vi "LVClass_SlopesPostProcessList dtor.vi"(0 "SlopesPostProcessorList in":refnum<class "SlopesPostProcessorList.lvclass">, 11 "error in (no error)":errorcluster) -> (4 "SlopesPostProcessorList out":refnum<class "SlopesPostProcessorList.lvclass">, 15 "error out":errorcluster)   [LabVIEW 2020, in "SlopesPostProcessorList.lvclass"]
doc: "SlopesPostProcessorList destructor.\n\n--------------------------------------------------------------------------------\n\n<B>SlopesPostProcessorListIn </B> : SlopesPostProcessorList object.\n<B>SlopesPostProcessorListOut </B> : SlopesPostProcessorList object.\n<B>ErrorIn </B> : Error\n<B>ErrorOut </B> : Error\n\n--------------------------------------------------------------------------------"
uses:
  SlopesPostProcessorList.lvclass
  SlopesPostProcessorList.lvclass/SlopesPostProcessorList.ctl
  HasoSlopes.lvclass
  Pupil.lvclass
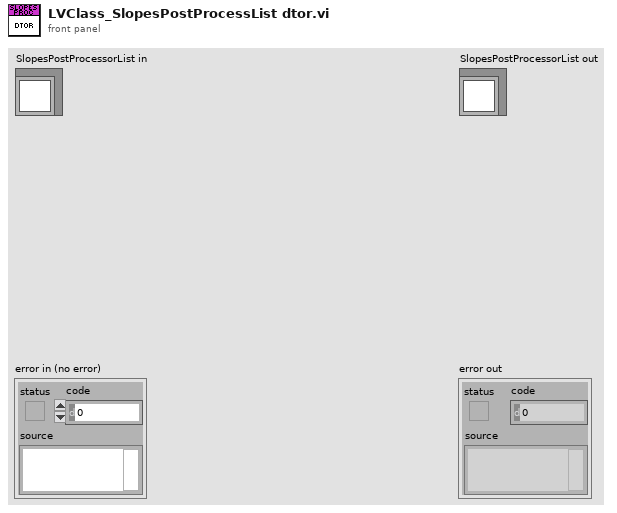
[diagram p1: front panel]
types:
  T1 = typedef "Handle creation.ctl" = enum16{"By ctor", "By write function"}
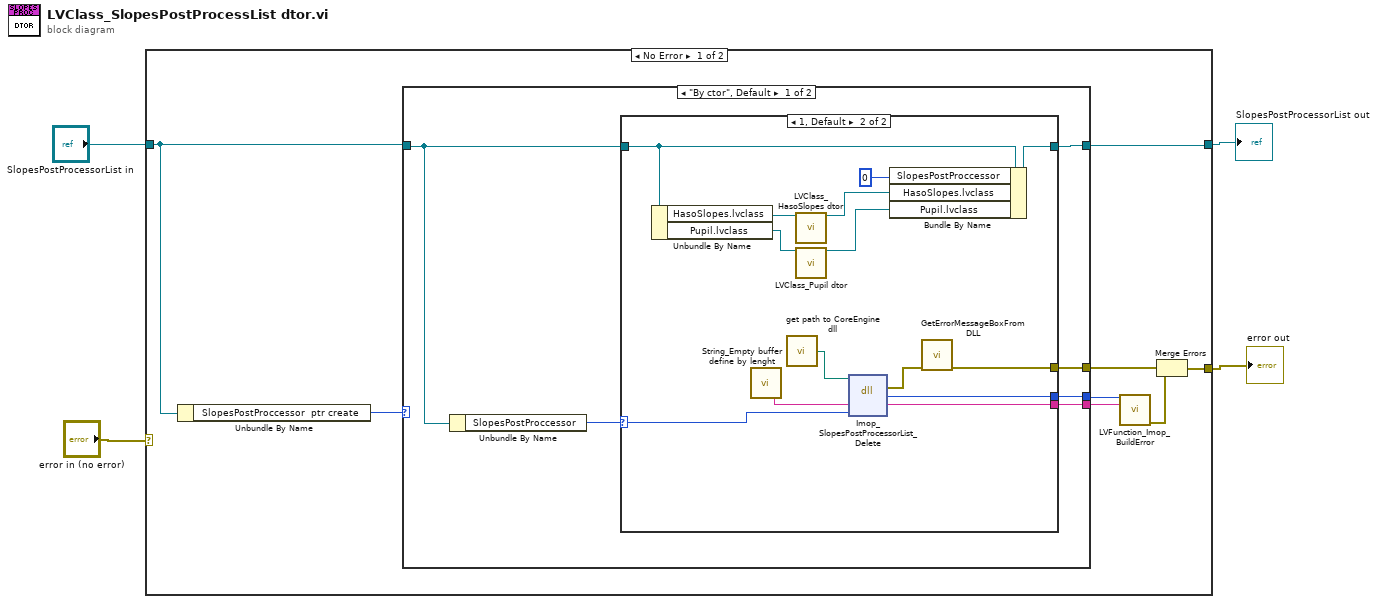
[diagram p0: block diagram]
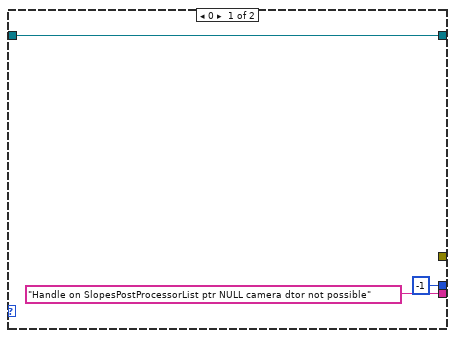
[diagram p2: hidden frame]
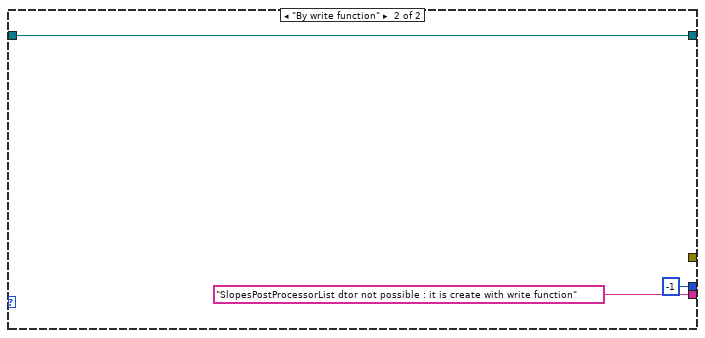
[diagram p3: hidden frame]
diagram:
  n1 = case shown="No Error" "error in (no error)" {
    selector: "error in (no error)" -> [_ w40]
    tunnel: [w5 w40] -> w2
    tunnel: [w10 w39] -> w1
    tunnel: "SlopesPostProcessorList in" -> [w9 w39]
    frame No Error {
      n2 = Unbundle By Name(w9) -> ("SlopesPostProccessor  ptr create"=w8:T1)
      n3 = case shown="\"By ctor\", Default" w8 {
        tunnel: [w18 w38] -> w10
        tunnel: [w17 -1] -> w12
        tunnel: [w16 "SlopesPostProcessorList dtor not possible : it is create with write function" ("message")] -> w11
        tunnel: w9 -> [w15 w38]
        tunnel: [w13 _] -> w7
        frame "By ctor", Default {
          n4 = Unbundle By Name(w15) -> ("SlopesPostProccessor"=w14:i32)
          n5 = case shown="1, Default" w14 {
            selector: w14 -> [_ w33]
            tunnel: w15 -> [w21 w27]
            tunnel: [w21 w35] -> w18
            tunnel: [-1 w31] -> w17
            tunnel: ["Handle on SlopesPostProcessorList ptr NULL camera dtor not possible" ("message") w32] -> w16
            tunnel: [_ w24] -> w13
            frame 0 {
            }
            frame 1, Default {
              n6 = Unbundle By Name(w27) -> ("HasoSlopes.lvclass"=w26:refnum<class "HasoSlopes.lvclass">, "Pupil.lvclass"=w25:refnum<class "Pupil.lvclass">)
              n7 = call "String_Empty buffer define by lenght.vi"() -> ("Empty buffer"=w34:string)  [unwired: 1 in]
              n8 = call "get path to CoreEngine dll.vi"() -> ("path to c_interface_vc100.dll"=w30:path)  [unwired: 12 in, 3 out]
              n9 = call "LVClass_HasoSlopes dtor.vi"("HasoSlopes in"=w26) -> ("HasoSlopes out"=w23:refnum<class "HasoSlopes.lvclass">)  [unwired: 13 in, 1 out]
              n10 = call "LVClass_Pupil dtor.vi"("Pupil in"=w25) -> ("Pupil out"=w22:refnum<class "Pupil.lvclass">)  [unwired: 13 in, 1 out]
              n11 = dll-call lib="D:/soft/HASO_v3/SVN_trunk/ImOpCoreEngine4_LV2011/DLLs/c_interface_vc100.dll" fn="Imop_SlopesPostProcessorList_Delete"(path in=w30, "message"=w34, "objet"=w33) -> (error out=w29:errorcluster, "return type"=w31:i32, "message"=w32:string)  [unwired: 3 in, 1 out]
              n12 = Bundle By Name(cluster=w27, "SlopesPostProccessor"=u32 0 ("Slope PPList"), "HasoSlopes.lvclass"=w23, "Pupil.lvclass"=w22) -> (w35:refnum<class "SlopesPostProcessorList.lvclass">)
              n13 = call "GetErrorMessageBoxFromDLL.vi"("error IN"=w29) -> ("error OUT"=w24:errorcluster)  [unwired: 10 in]
            }
          }
        }
        frame "By write function" {
        }
      }
      n14 = call "LVFunction_Imop_BuildError.vi"("code"=w12, "String to Prepend to source (\"\")"=w11) -> ("error out"=w6:errorcluster)  [unwired: 13 in]
      n15 = Merge Errors(w7, w6) -> (w5:errorcluster)
    }
    frame Error {
    }
  }
  "error out" <- w2
  "SlopesPostProcessorList out" <- w1
